vi "LookupFormatConfig.vi"(11 "format string":string) -> (3 "Formatter Config out":refnum<class "Formatter Config.lvclass">)   [LabVIEW 2015]
uses:
  Report Formatters/Base Class/Config/Formatter Config.lvclass
  Report Formatters/csv/Config/csv-formatter Config.lvclass
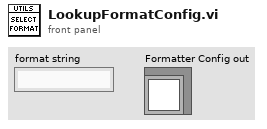
[diagram p1: front panel]
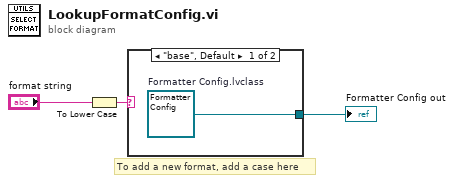
[diagram p0: block diagram]
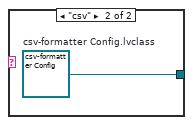
[diagram p2: hidden frame]
diagram:
  # "To add a new format, add a case here"
  n1 = To Lower Case(string="format string") -> (all lower case string=w3:string)
  n2 = case shown="\"base\", Default" w3 {
    tunnel: [w4 w5] -> w1
    frame "base", Default {
      w4 = refnum<class "Formatter Config.lvclass"> refnum  # Formatter Config.lvclass
    }
    frame "csv" {
      w5 = refnum<class "csv-formatter Config.lvclass"> refnum  # csv-formatter Config.lvclass
    }
  }
  "Formatter Config out" <- w1
